vi "GlobalCostants.vi"() -> ()   [LabVIEW 2010]
uses:
  VarableStruct.ctl
  VarableID.ctl
panel:
  in  "PortIPList":string[](array[string])
  in  "CommandCodeList":cluster{"CommandCode":string, "VarableID":T1}[](array[cluster])
  in  "VarableList":T2[](array[typedef])
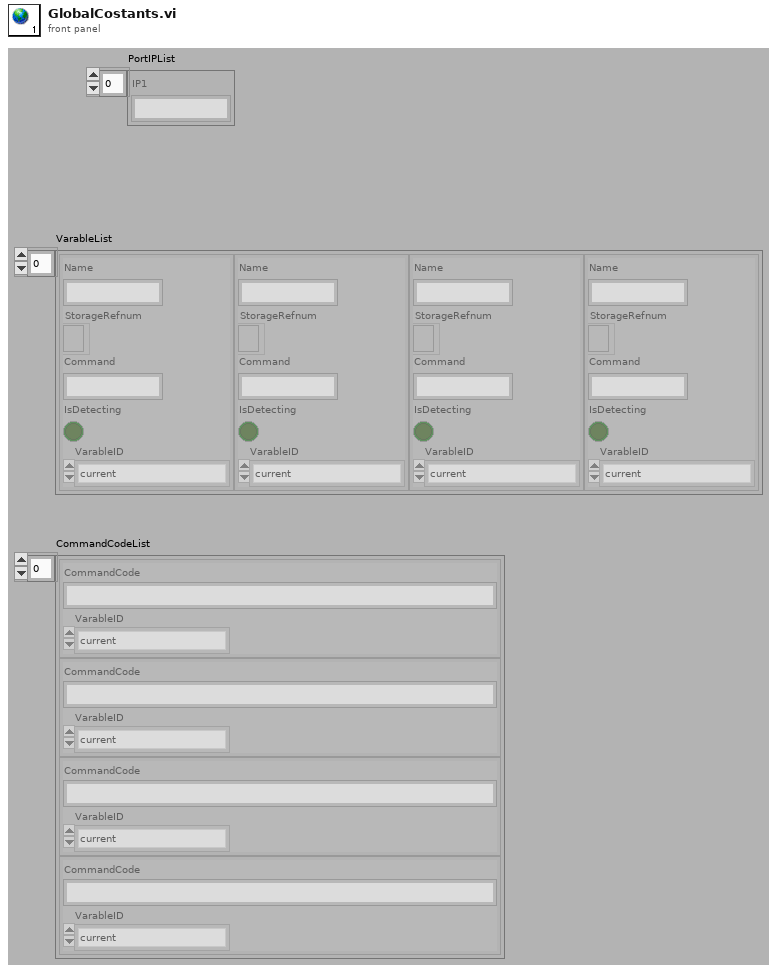
[diagram p1: front panel]
types:
  T1 = typedef "VarableID.ctl" = enum16{"current", "voltage", "power", "PF"}
  T2 = typedef "VarableStruct.ctl" = cluster{"Name":string, "StorageRefnum":refnum<file>, "Command":string, "IsDetecting":bool, "VarableID":T1}
diagram:
